vi "Eat.vi"(8 "error in (no error)":errorcluster caption="错误输入（无错误）", 10 "字符串":string, 11 "eagle 输入":refnum<class "eagle.lvclass">) -> (0 "error out":errorcluster caption="错误输出", 2 "字符串 2":string, 3 "eagle 输出":refnum<class "eagle.lvclass">)   [LabVIEW 2020, in "eagle.lvclass"]
uses:
  eagle.lvclass
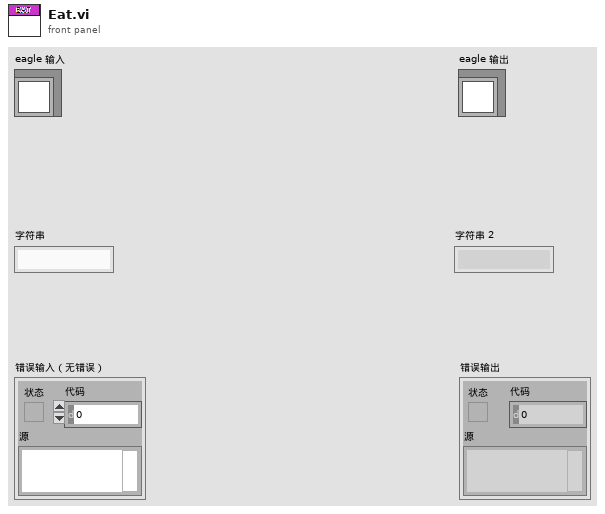
[diagram p1: front panel]
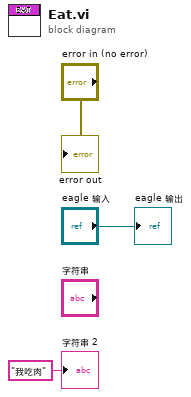
[diagram p0: block diagram]
diagram:
  "error out" <- "error in (no error)"
  "eagle 输出" <- "eagle 输入"
  "字符串 2" <- "我吃肉" ("字符串 2")
